vi "Semi Active Scheduler Engine.vi"(8 "Number of  Jobs":i32=4, 9 "Number of Machines":i32=4, 10 "Processing Times":u16[][](array[numeric])=[[34, 15, 38, 95], [2, 89, 19, 7], [54, 70, 28, 34], [61, 9, 87, 29]], 11 "Schedule":u16[](array[numeric])=[12, 0, 7, 2, 6, 3, 13, 5, 1, 4, 14, 11, 10, 15, 8, 9]) -> (0 "Reordered Schedule Out":u16[](array[numeric]), 1 "Job Completion Times":u16[](array[numeric]), 2 "Completion Times":u16[][](array[numeric]), 3 "Start Times":u16[][](array[numeric]), 4 "Machine Completion Times":u16[](array[numeric]))   [LabVIEW 2013, in "Scheduler.lvclass"]
uses:
  Scheduler.lvclass
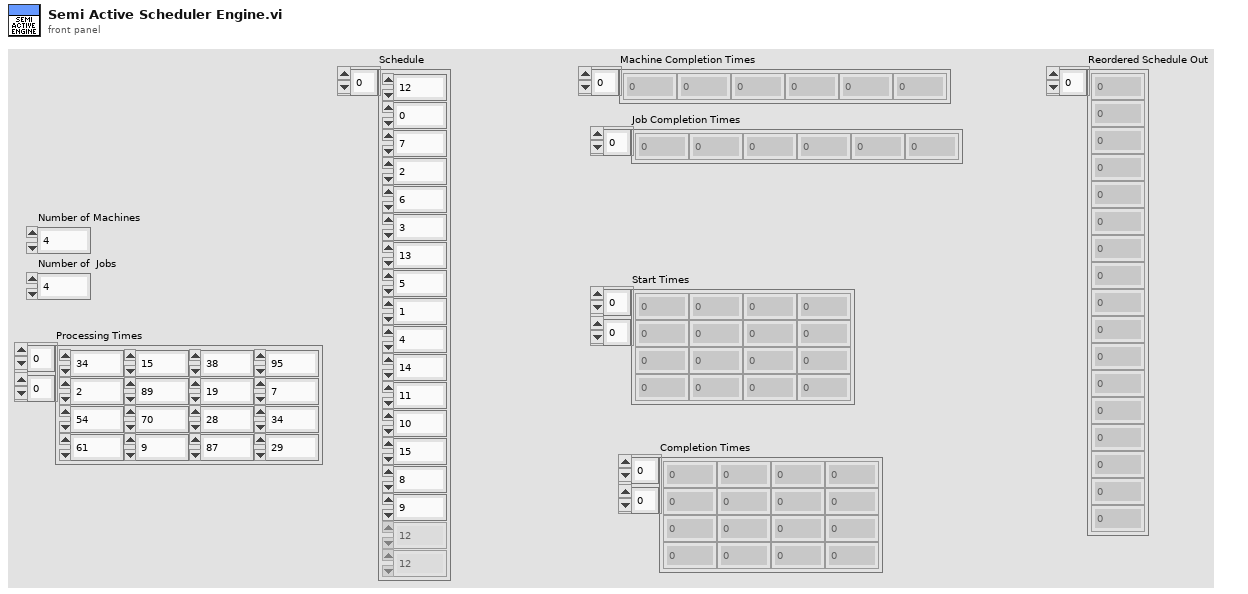
[diagram p1: front panel]
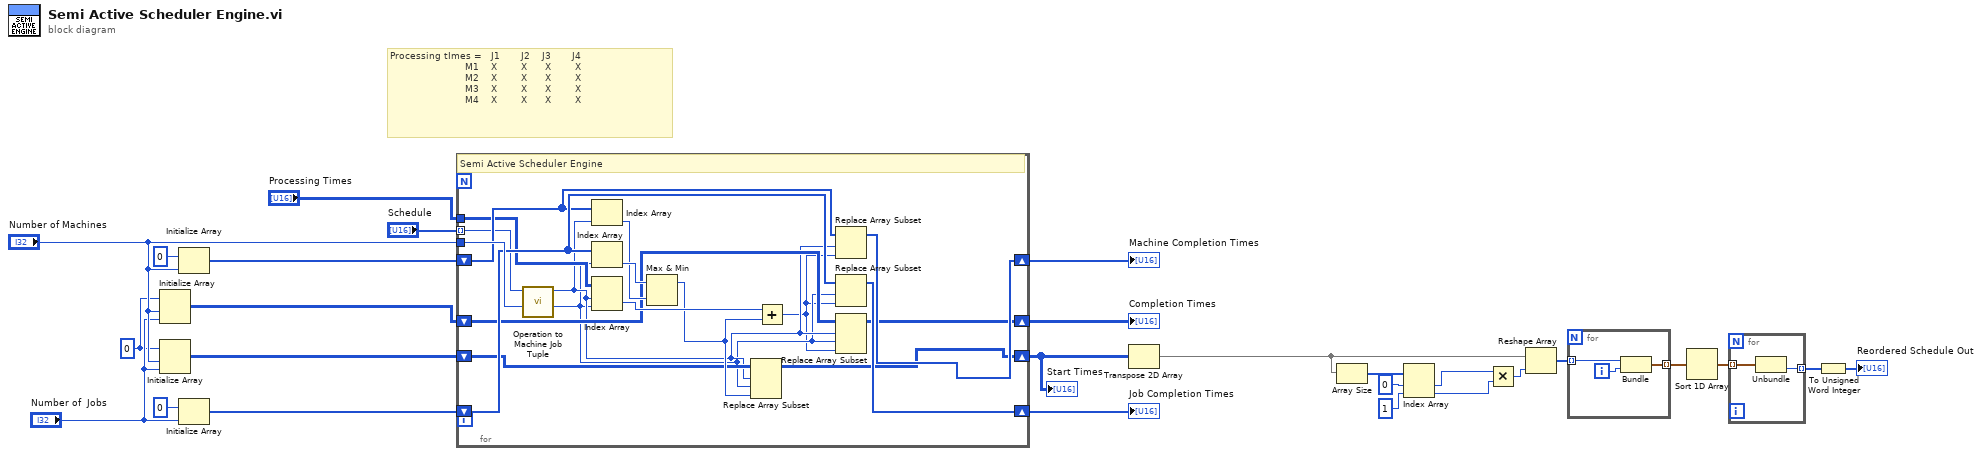
[diagram p0: block diagram]
diagram:
  w15 = u16 0 ("element")
  # "Processing tImes =   J1       J2    J3       J4   \n                         M1    X        X      X        X\n                         M2    X        X      X        X\n                         M3    X        X      X        X\n                         M4    X        X      X        X"
  n1 = Initialize Array(w15, "Number of Machines", "Number of  Jobs") -> (w22:u16[][])
  n2 = Initialize Array(w15, "Number of Machines", "Number of  Jobs") -> (w14:u16[][])
  n3 = Initialize Array(u16 0 ("element"), "Number of Machines") -> (w24:u16[])
  n4 = Initialize Array(u16 0 ("element"), "Number of  Jobs") -> (w25:u16[])
  n5 = for {
    tunnel: "Number of Machines" -> [w45]
    shift-right: [w42] -> w20
    shift-left: w25 -> [w44]
    shift-right: [w41] -> w19
    shift-left: w24 -> [w43]
    shift-right: [w28] -> w21
    shift-left: w22 -> [w32]
    tunnel: "Processing Times" -> [w40]
    shift-right: [w33] -> w2
    shift-left: w14 -> [w34]
    tunnel: "Schedule" -> [w38] mode=indexing
    # "Semi Active Scheduler Engine"
    n6 = call "Operation to Machine Job Tuple.vi"("Number of Machines"=w45, "Operation Number"=w38) -> ("Job No"=w30:i32, "Machine No"=w31:i32)  [unwired: 8 in]
    n7 = Index Array(array=w43, index=w31) -> (element=w36:u16)
    n8 = Index Array(array=w44, index=w30) -> (element=w37:u16)
    n9 = Index Array(array=w40, index (row)=w31, index (col)=w30) -> (element=w39:u16)
    n10 = Max & Min(x=w37, y=w36) -> (max(x,y)=w35:u16)  [unwired: 1 out]
    n11 = Replace Array Subset(array=w34, new element=w35, index (row)=w31, index (col)=w30) -> (w33:u16[][])
    n12 = Add(x=w39, y=w35) -> (x+y=w29:u16)
    n13 = Replace Array Subset(array=w43, new element=w29, index=w31) -> (w41:u16[])
    n14 = Replace Array Subset(array=w44, new element=w29, index=w30) -> (w42:u16[])
    n15 = Replace Array Subset(array=w32, new element=w29, index (row)=w31, index (col)=w30) -> (w28:u16[][])
  }
  "Completion Times" <- w21
  "Job Completion Times" <- w20
  "Machine Completion Times" <- w19
  "Start Times" <- w2
  n16 = Transpose 2D Array(2D array=w2) -> (transposed array=w8:u16[][])
  n17 = Array Size(array=w8) -> (size(s)=w13:i32[])
  n18 = Index Array(array=w13, index #1=0 ("index"), index #2=1 ("index")) -> (element #1=w10:i32, element #2=w9:i32)
  n19 = Multiply(x=w10, y=w9) -> (x*y=w7:i32)
  n20 = Reshape Array(w8, w7) -> (w6:u16[])
  n21 = for {
    tunnel: w6 -> [w48] mode=indexing
    tunnel: [w46] -> w5 mode=indexing
    i -> [w47]
    n22 = Bundle("element"=w48, w47) -> (w46:cluster{"element":u16, i32})  [unwired: 1 in]
  }
  n23 = Sort 1D Array(array=w5) -> (sorted array=w4:cluster{"element":u16, i32}[])
  n24 = for {
    tunnel: w4 -> [w50] mode=indexing
    tunnel: [w49] -> w3 mode=indexing
    n25 = Unbundle(w50) -> (w49:i32)  [unwired: 1 out]
  }
  n26 = To Unsigned Word Integer(number=w3) -> (unsigned 16bit integer=→"Reordered Schedule Out":u16[])
